vi "OverWritingConfig.vi"(10 "NewVal":T1, 11 "local path":path) -> (3 "Refnum out":T2)   [LabVIEW 2014]
uses:
  <vilib>/Utility/config.llb/Config Data RefNum.ctl
  <vilib>/Utility/config.llb/Write Key (Double).vi
  <vilib>/Utility/config.llb/NI_LVConfig.lvlib
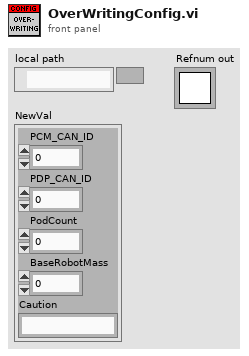
[diagram p1: front panel]
types:
  T1 = cluster{"PCM_CAN_ID":dbl, "PDP_CAN_ID":dbl, "PodCount":dbl, "BaseRobotMass":dbl, "Caution":string}
  T2 = typedef "NI_LVConfig.lvlib/Config Data RefNum.ctl" = refnum<k1>
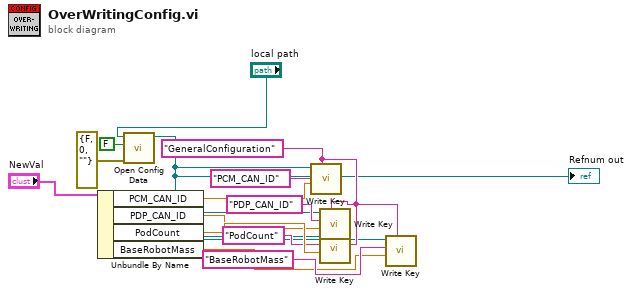
[diagram p0: block diagram]
diagram:
  w12 = "GeneralConfiguration" ("name or relative path")
  n1 = Unbundle By Name("NewVal") -> ("PCM_CAN_ID"=w7:dbl, "PDP_CAN_ID"=w9:dbl, "PodCount"=w11:dbl, "BaseRobotMass"=w13:dbl)
  n2 = call <vilib>:"Open Config Data.vi"("error in (no error)"=errorcluster {"status"=FALSE, "code"=0, "source"=""}, "create file if necessary (T)"=FALSE, "configuration file path"="local path") -> ("refnum"=w3:T2)  [unwired: 6 in, 2 out]
  "Refnum out" <- w3
  n3 = call-poly <vilib>:"Write Key.vi"("section"=w12, "value"=w7, "key"="PCM_CAN_ID" ("string"), "refnum"=w3) -> ()  [unwired: 5 in, 3 out]
  n4 = call-poly <vilib>:"Write Key.vi"("section"=w12, "value"=w9, "key"="PDP_CAN_ID" ("string"), "refnum"=w3) -> ()  [unwired: 5 in, 3 out]
  n5 = call-poly <vilib>:"Write Key.vi"("section"=w12, "value"=w11, "key"="PodCount" ("string"), "refnum"=w3) -> ()  [unwired: 5 in, 3 out]
  n6 = call-poly <vilib>:"Write Key.vi"("section"=w12, "value"=w13, "key"="BaseRobotMass" ("string"), "refnum"=w3) -> ()  [unwired: 5 in, 3 out]
